vi "WriteToDictionary.vi"(7 "Qualified Name":string[](array[string]), 8 "error in (no error)":errorcluster, 9 "Values":string[](array[string]), 10 "Keys":string[](array[string]), 11 "ConfigManager.Text in":refnum<class "ConfigManager.Text.lvclass">) -> (0 "error out":errorcluster, 3 "ConfigManager.Text out":refnum<class "ConfigManager.Text.lvclass">)   [LabVIEW 2013, in "CfgManager.Text.lvlib" / "ConfigManager.Text.lvclass"]
uses:
  ConfigManager.Text.lvclass
  ConfigManager.Text.lvclass/ConfigManager.Text.ctl
  <vilib>/LabVIEW Open Source Project/Unicity/Delimiter/Delimiter.lvclass
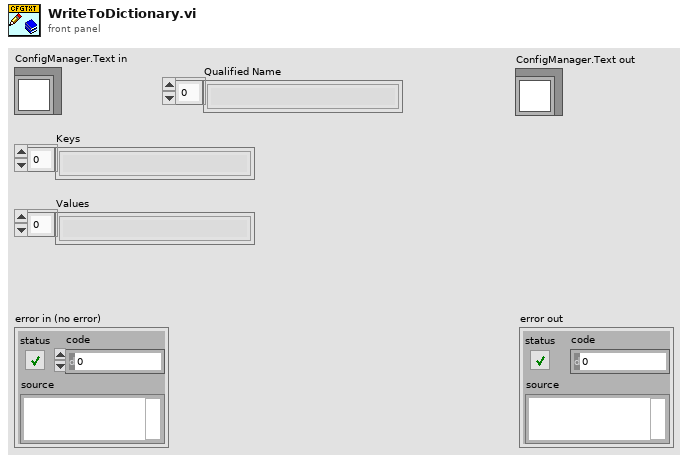
[diagram p1: front panel]
types:
  T1 = typedef "CfgManager.Text.lvlib/ConfigManager.Text.lvclass/Configuration -- Cluster.ctl" = cluster{"FileHeader":refnum<class "FileHeader.lvclass">, "FileSignature":refnum<class "FileSignature.lvclass">, "Section Delimiter":refnum<class "Delimiter.lvclass">, "Key-Value Separator":refnum<class "Delimiter.lvclass">}
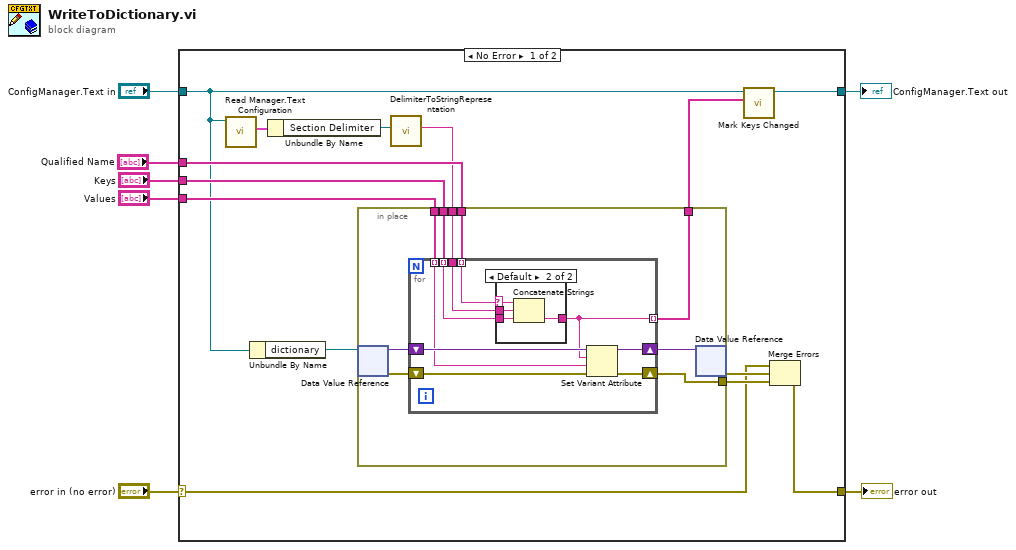
[diagram p0: block diagram]
diagram:
  n1 = case shown="No Error" "error in (no error)" {
    selector: "error in (no error)" -> [w16 w46]
    tunnel: [w21 w46] -> w7
    tunnel: "Values" -> [w18 _]
    tunnel: "Keys" -> [w13 _]
    tunnel: "ConfigManager.Text in" -> [w8 w45]
    tunnel: [w10 w45] -> w2
    tunnel: "Qualified Name" -> [w12 _]
    frame No Error {
      n2 = call "Read Manager.Text Configuration.vi"("ConfigManager.Text in"=w8) -> ("Manager.Text Configuration"=w14:T1)  [unwired: 9 in, 1 out]
      n3 = Unbundle By Name(w8) -> ("dictionary"=w17:refnum<data-value>)
      n4 = Unbundle By Name(w14) -> ("Section Delimiter"=w15:refnum<class "Delimiter.lvclass">)
      n5 = call <vilib>:"DelimiterToStringRepresentation.vi"("Delimiter"=w15) -> ("String representation"=w11:string)  [unwired: 10 in]
      n6 = in-place {
        in-place-border: w13 -> [w28]
        in-place-border: w18 -> [w27]
        in-place-border: [w25] -> w20
        in-place-border: w12 -> [w24]
        in-place-border: w11 -> [w23]
        in-place-border: [w22] -> w9
        n7 = in-place-dvr #1(w17) -> (w30:variant, w26:errorcluster)
        n8 = for {
          shift-right: [w38] -> w29
          shift-left: w30 -> [w39]
          tunnel: w28 -> [w32] mode=indexing
          tunnel: w27 -> [w35] mode=indexing
          shift-right: [w36] -> w25
          shift-left: w26 -> [w37]
          tunnel: w24 -> [w34] mode=indexing
          tunnel: w23 -> [w33]
          tunnel: [w31] -> w22 mode=indexing
          n9 = case shown="Default" w34 {
            selector: w34 -> [_ w41]
            tunnel: w32 -> [w40 w44]
            tunnel: [w40 w43] -> w31
            tunnel: w33 -> [_ w42]
            frame "" {
            }
            frame Default {
              n10 = Concatenate Strings(w41, w42, w44) -> (w43:string)
            }
          }
          n11 = Set Variant Attribute(Variant=w39, name=w31, value=w35, error in=w37) -> (Variant out=w38:variant, error out=w36:errorcluster)  [unwired: 1 out]
        }
        n12 = in-place-dvr #1(w29) -> (w19:errorcluster)  [unwired: 1 out]
      }
      n13 = call "Mark Keys Changed.vi"("Changed keys"=w9, "ConfigManager.Text in"=w8) -> ("ConfigManager.Text out"=w10:refnum<class "ConfigManager.Text.lvclass">)  [unwired: 9 in]
      n14 = Merge Errors(w16, w19, w20) -> (w21:errorcluster)
    }
    frame Error {
    }
  }
  "error out" <- w7
  "ConfigManager.Text out" <- w2
